vi "DSF.Shared.Timing.Set Offset.vi"(10 "Offset":u64, 11 "Timing in":refnum<class "DSF.Shared.Timing.lvclass">) -> (3 "Timing out":refnum<class "DSF.Shared.Timing.lvclass">)   [LabVIEW 2017, in "DSF.Shared.lvlib" / "DSF.Shared.Timing.lvclass"]
uses:
  DSF.Shared.Timing.lvclass
  DSF.Shared.Timing.lvclass/DSF.Shared.Timing.ctl
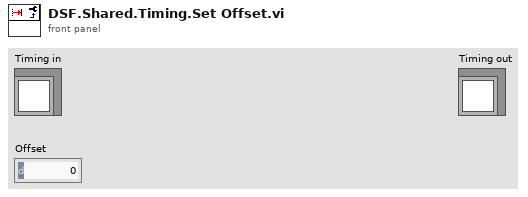
[diagram p1: front panel]
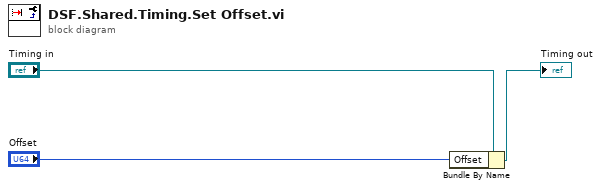
[diagram p0: block diagram]
diagram:
  n1 = Bundle By Name(cluster="Timing in", "Offset"="Offset") -> (→"Timing out":refnum<class "DSF.Shared.Timing.lvclass">)
